vi "RPC Extended Core.vi"(0 "TwinCAT ADS in":refnum<class "TwinCAT ADS.lvclass">, 2 "Type":variant, 5 "Name":string, 7 "Method":string, 9 "Parameters":variant[](array[variant]), 11 "error in (no error)":errorcluster) -> (4 "TwinCAT ADS out":refnum<class "TwinCAT ADS.lvclass">, 10 "Value":variant, 15 "error out":errorcluster)   [LabVIEW 2018, in "TwinCAT ADS.lvclass"]
uses:
  TwinCAT ADS.lvclass
  TwinCAT.Ads
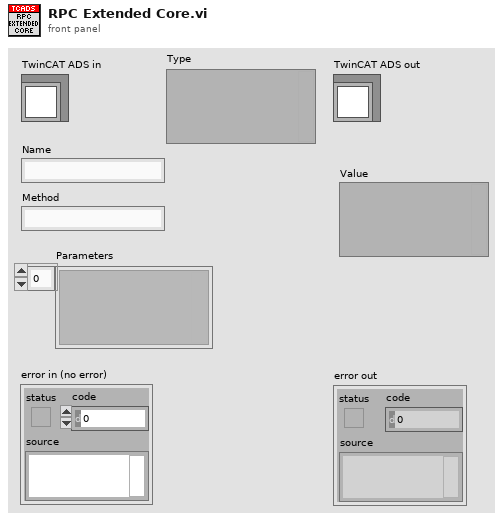
[diagram p1: front panel]
types:
  T1 = typedef "TwinCAT ADS.lvclass/Method Information.ctl" = cluster{"Name":string, "Parameters":T2[], "Parameter Count":i32, "Is Void?":bool, "Return Type":string, "Return Type Size":i32, "Comment":string}
  T2 = typedef "TwinCAT ADS.lvclass/Method Parameter Information.ctl" = cluster{"Name":string, "Type Name":string, "Size":i32, "Parameter Flags":u32, "Has LengthIs Parameter?":bool, "LengthIs Parameter Index":i32}
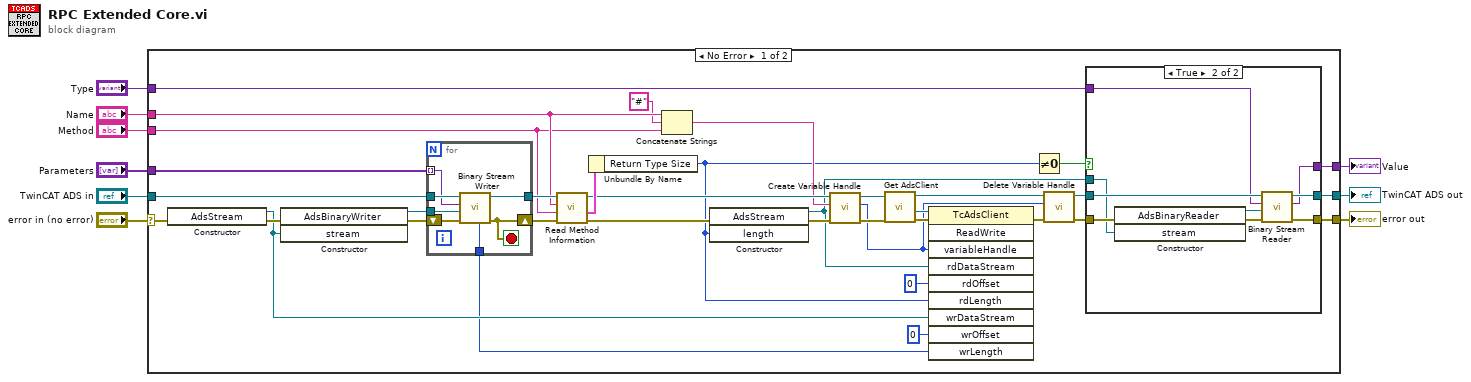
[diagram p0: block diagram]
diagram:
  n1 = case shown="No Error" "error in (no error)" {
    selector: "error in (no error)" -> [w42 w65]
    tunnel: [w11 w65] -> w8
    tunnel: [w12 w64] -> w6
    tunnel: "TwinCAT ADS in" -> [w41 w64]
    tunnel: "Parameters" -> [w40 _]
    tunnel: "Method" -> [w34 _]
    tunnel: "Name" -> [w35 _]
    tunnel: "Type" -> [w17 _]
    tunnel: [w10 _] -> w1
    frame No Error {
      n2 = constructor class="AdsStream"(error in=w42) -> (reference out=w21:refnum<k24>, error out=w45:errorcluster)  [unwired: 2 in, 1 out]
      n3 = constructor class="AdsBinaryWriter"(error in=w45, "stream"=w21) -> (reference out=w43:refnum<k24>, error out=w44:errorcluster)  [unwired: 2 in, 2 out]
      n4 = for {
        tunnel: w43 -> [w62]
        tunnel: w41 -> [w61]
        tunnel: w40 -> [w60] mode=indexing
        tunnel: [w59] -> w38
        shift-right: [w58] -> w39
        shift-left: w44 -> [w63]
        tunnel: [w57] -> w20
        stop <- w58 stop-if-true
        n5 = call "Binary Stream Writer.vi"("error in (no error)"=w63, ".NET AdsBinaryWriter refnum"=w62, "Value"=w60, "TwinCAT ADS in"=w61) -> ("error out"=w58:errorcluster, "TwinCAT ADS out"=w59:refnum<class "TwinCAT ADS.lvclass">, "Length"=w57:i64)  [unwired: 4 in, 1 out]
      }
      n6 = call-dynamic "Read Method Information.vi"("error in (no error)"=w39, "Method"=w34, "Name"=w35, "TwinCAT ADS in"=w38) -> ("error out"=w37:errorcluster, "Method Information"=w36:T1, "TwinCAT ADS out"=w31:refnum<class "TwinCAT ADS.lvclass">)  [unwired: 5 in]
      n7 = Unbundle By Name(w36) -> ("Return Type Size"=w14:i32)
      n8 = Concatenate Strings(w35, "#" ("string"), w34) -> (w30:string)
      n9 = constructor class="AdsStream"(error in=w37, "length"=w14) -> (reference out=w15:refnum<k24>, error out=w32:errorcluster)  [unwired: 2 in, 2 out]
      n10 = call-dynamic "Create Variable Handle.vi"("error in (no error)"=w32, "Name"=w30, "TwinCAT ADS in"=w31) -> ("error out"=w27:errorcluster, "Handle"=w23:i32, "TwinCAT ADS out"=w26:refnum<class "TwinCAT ADS.lvclass">)  [unwired: 6 in]
      n11 = call-dynamic "Get AdsClient.vi"("error in (no error)"=w27, "TwinCAT ADS in"=w26) -> ("error out"=w29:errorcluster, ".NET TcAdsClient refnum"=w28:refnum<k24>, "TwinCAT ADS out"=w24:refnum<class "TwinCAT ADS.lvclass">)  [unwired: 7 in]
      n12 = invoke class="TcAdsClient" method="ReadWrite"(reference=w28, error in=w29, "variableHandle"=w23, "rdDataStream"=w15, "rdOffset"=0, "rdLength"=w14, "wrDataStream"=w21, "wrOffset"=0, "wrLength"=w20) -> (error out=w25:errorcluster)  [unwired: 1 in, 9 out]
      n13 = Not Equal To 0?(x=w14) -> (x != 0?=w13:bool)
      n14 = call-dynamic "Delete Variable Handle.vi"("error in (no error)"=w25, "Handle"=w23, "TwinCAT ADS in"=w24) -> ("error out"=w16:errorcluster, "TwinCAT ADS out"=w18:refnum<class "TwinCAT ADS.lvclass">)  [unwired: 7 in]
      n15 = case shown="True" w13 {
        tunnel: w18 -> [w46 w56]
        tunnel: w17 -> [_ w55]
        tunnel: w16 -> [w47 w54]
        tunnel: w15 -> [_ w53]
        tunnel: [w47 w50] -> w11
        tunnel: [w46 w49] -> w12
        tunnel: [_ w48] -> w10
        frame False {
        }
        frame True {
          n16 = constructor class="AdsBinaryReader"(error in=w54, "stream"=w53) -> (reference out=w51:refnum<k24>, error out=w52:errorcluster)  [unwired: 2 in, 2 out]
          n17 = call "Binary Stream Reader.vi"("error in (no error)"=w52, ".NET AdsBinaryReader refnum"=w51, "Type"=w55, "TwinCAT ADS in"=w56) -> ("error out"=w50:errorcluster, "Value"=w48:variant, "TwinCAT ADS out"=w49:refnum<class "TwinCAT ADS.lvclass">)  [unwired: 4 in, 1 out]
        }
      }
    }
    frame Error {
    }
  }
  "error out" <- w8
  "TwinCAT ADS out" <- w6
  "Value" <- w1
